vi "Message Read Loop.vi"(8 "error in (no error)":errorcluster, 11 "Actor in":refnum<class "Actor.lvclass">) -> (0 "error out":errorcluster, 3 "Actor out":refnum<class "Actor.lvclass">)   [LabVIEW 2022 SP3, in "Artifex.lvlib" / "Actor.lvclass"]
uses:
  Actor.lvclass
  Actor Proxy/Actor API.lvclass/Actor API.ctl
  Priority Message Queue/Priority Dequeue.vi
  Actor Proxy/Stop Nested.vi
  Actor Proxy/Actor API.lvclass
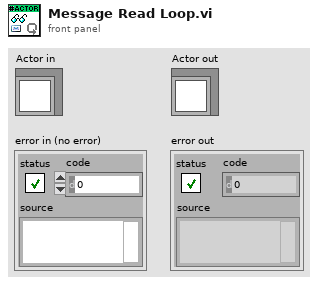
[diagram p1: front panel]
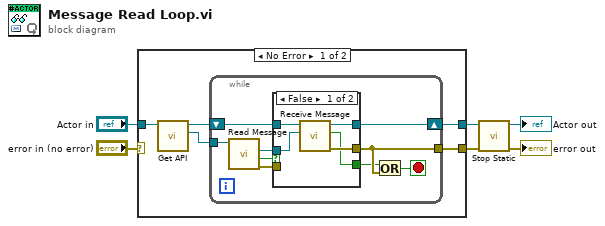
[diagram p0: block diagram]
diagram:
  n1 = case shown="No Error" "error in (no error)" {
    selector: "error in (no error)" -> [_ w29]
    tunnel: "Actor in" -> [w11 w28]
    tunnel: [w10 w28] -> w4
    tunnel: [w9 w29] -> w3
    frame No Error {
      n2 = call-dynamic "Get API.vi"("Actor in"=w11) -> ("Actor API"=w7:refnum<class "Actor API.lvclass">, "Actor out"=w8:refnum<class "Actor.lvclass">)  [unwired: 8 in, 1 out]
      n3 = while {
        tunnel: w7 -> [w20]
        shift-right: [w16] -> w10
        shift-left: w8 -> [w17]
        tunnel: [w14] -> w9
        stop <- w12 stop-if-true
        n4 = call "Read Message.vi"("Actor API in"=w20) -> ("error out"=w15:errorcluster, "Timeout"=w19:bool, "Message"=w18:refnum<class "Message.lvclass">)  [unwired: 7 in, 1 out]
        n5 = case shown="False" w19 {
          tunnel: w18 -> [w23 _]
          tunnel: w17 -> [w25 w27]
          tunnel: [w24 w27] -> w16
          tunnel: w15 -> [_ w26]
          tunnel: [w22 w26] -> w14
          tunnel: [w21 _] -> w13
          frame False {
            n6 = call-dynamic "Receive Message.vi"("Message"=w23, "Actor in"=w25) -> ("error out"=w22:errorcluster, "Stop Actor"=w21:bool, "Actor out"=w24:refnum<class "Actor.lvclass">)  [unwired: 7 in]
          }
          frame True {
          }
        }
        n7 = Or(x=w13, y=w14) -> (x .or. y?=w12:bool)
      }
    }
    frame Error {
    }
  }
  n8 = call "Stop Static.vi"("error in (no error)"=w3, "Actor in"=w4) -> ("error out"=→"error out":errorcluster, "Actor out"=→"Actor out":refnum<class "Actor.lvclass">)  [unwired: 8 in]
